vi "avi capture example.vi"() -> ()   [LabVIEW 2009]
uses:
  <vilib>/userDefined/High Color/IMAQdx.ctl
  <vilib>/vision/driver/IMAQdx.llb/IMAQdx Camera Control Mode.ctl
  <vilib>/vision/driver/NI_Vision_Acquisition_Software.lvlib
panel:
  in  "AVI Path":path
  out "Image":T1(plugin-control)
  in  "stop":bool
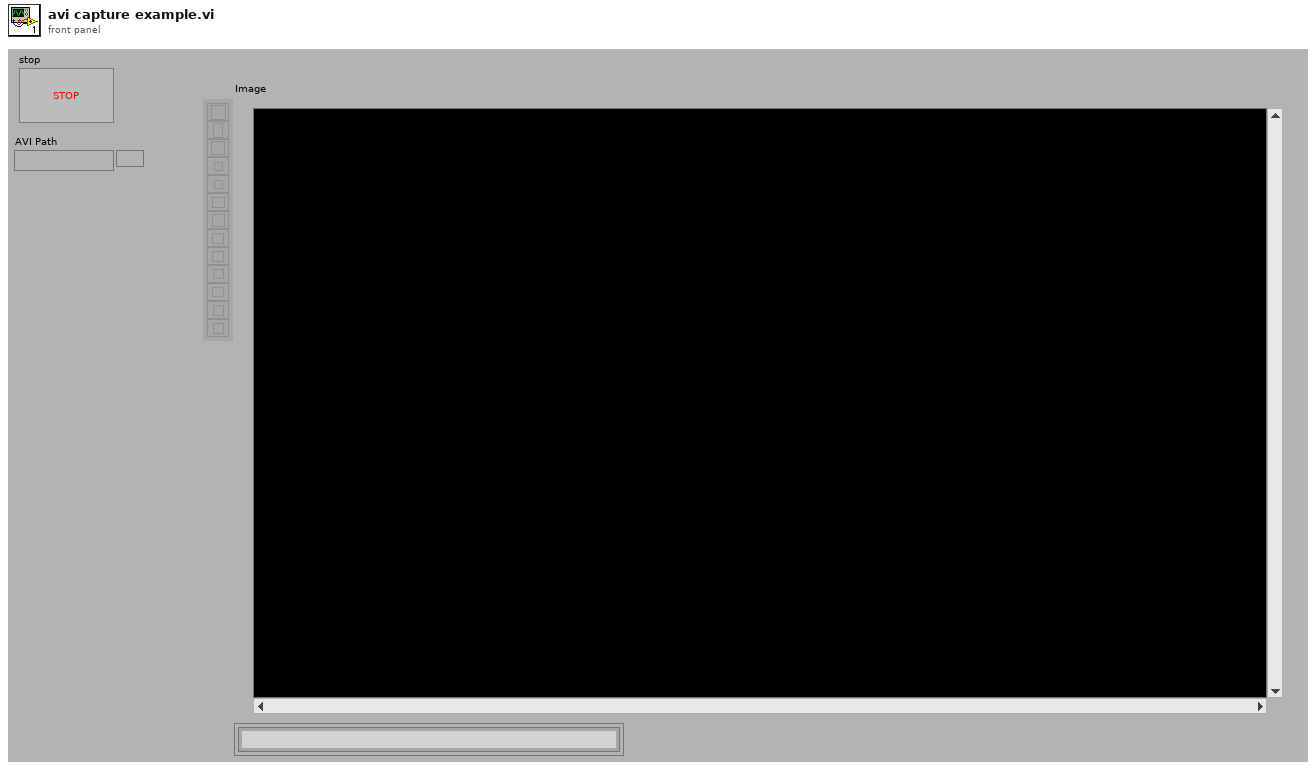
[diagram p1: front panel]
types:
  T1 = typedef "IMAQ Image.ctl" = refnum<image>
  T2 = typedef "NI_Vision_Acquisition_Software.lvlib/IMAQdx Camera Control Mode.ctl" = enum32{"Controller", "Listener"}
  T3 = typedef "IMAQdx.ctl" = refnum<k21>
  T4 = typedef "AviRefnum.ctl" = refnum<k1>
  T5 = typedef "Image Type" = u32
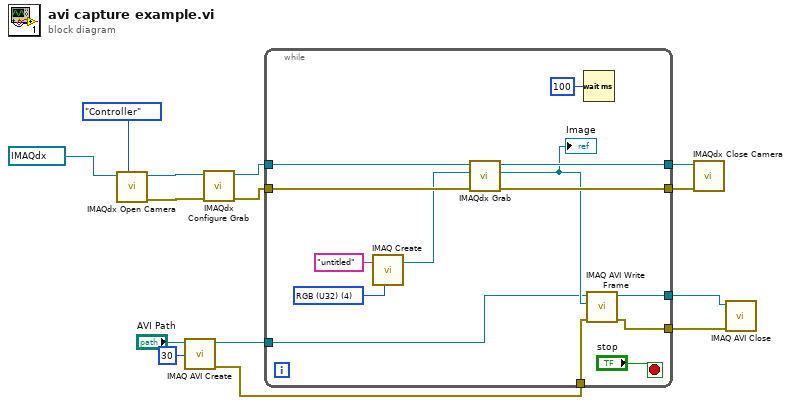
[diagram p0: block diagram]
diagram:
  n1 = call <vilib>:"IMAQdx Open Camera.vi"("Camera Control Mode"=IMAQdx_Camera_Control_Mode."Controller", "Session In"=T3 "cam1") -> ("error out"=w1:errorcluster, "Session Out"=w2:T3)  [unwired: 8 in]
  n2 = call "IMAQ AVI Create"("Frames Per Second"=u32 30, "AVI Path"="AVI Path") -> ("error out"=w9:errorcluster, "Avi Refnum"=w10:T4)  [unwired: 8 in]
  n3 = call <vilib>:"IMAQdx Configure Grab.vi"("error in"=w1, "Session In"=w2) -> ("error out"=w3:errorcluster, "Session Out"=w4:T3)  [unwired: 8 in]
  n4 = while {
    tunnel: [w27] -> w14
    tunnel: [w26] -> w13
    tunnel: w4 -> [w16]
    tunnel: w3 -> [w25]
    tunnel: w10 -> [w20]
    tunnel: w9 -> [w19]
    tunnel: [w18] -> w8
    tunnel: [w17] -> w7
    stop <- "stop" stop-if-true
    w22 = T5 4 items=["Grayscale (U8)", "Grayscale (I16)", "Grayscale (SGL)", "Complex (CSG)", "RGB (U32)", "HSL (U32)", "RGB (U64)", "Grayscale (U16)"] ("Image Type")
    n5 = call "IMAQ Create"("Image Name"="untitled", "Image Type"=w22) -> ("New Image"=w24:T1)  [unwired: 3 in, 1 out]
    n6 = call <vilib>:"IMAQdx Grab.vi"("error in"=w25, "Image In"=w24, "Session In"=w16) -> ("error out"=w26:errorcluster, "Image Out"=w21:T1, "Session Out"=w27:T3)  [unwired: 5 in, 1 out]
    "Image" <- w21
    n7 = Wait (ms)(milliseconds to wait=u32 100) -> ()  [unwired: 1 out]
    n8 = call "IMAQ AVI Write Frame"("error in (no error)"=w19, "Image"=w21, "Avi Refnum"=w20) -> ("error out"=w18:errorcluster, "Avi Refnum (duplicate)"=w17:T4)  [unwired: 7 in]
  }
  n9 = call <vilib>:"IMAQdx Close Camera.vi"("error in"=w13, "Session In"=w14) -> ()  [unwired: 9 in, 1 out]
  n10 = call "IMAQ AVI Close"("error in (no error)"=w8, "Avi Refnum"=w7) -> ()  [unwired: 9 in, 1 out]
